vi "Empty_Complete.vi"(11 "input cluster":T1={"Pinch-valve"="Test Sample", "XLP 6000 Pump"="MRJ", "Camera1"="", "Camera2"="", "Img_Capt"=FALSE, "Actuator"=FALSE, "Pump"=FALSE, "Cam 1"=FALSE, "Cam 2"=FALSE, "Empty_Refill"=FALSE, "Crop"=FALSE, "Light intensity"=0, "Exposure Time"=0.0, "Sample Name"="", "Operator"="", "Calibration 1"=path "C:/Users/au540322/Desktop/IHS_Project/images/Debris/Debris_0/Debris_0_2019_06_01-23-32-49-686.PNG", "Calibration 2"=path "C:/Users/au540322/Desktop/IHS_Project/images/Debris/Debris_0/Debris_0_2019_06_01-23-32-49-686.PNG", "Framerate"=1, "Timeout Sample"=1, "Collection date"="", "Sample size threshold"=500, "Empty start"=500, "Command"="", "Station"="", "Species Name"="", "Other Notes"="", "Aperture"=enum."Item 3", "Image Process Queue Size"=100, "Image Save Queue Size"=0, "Overload threshold"=0, "Max Framerate"=0, "Rectangle 1"={"Left"=0, "Top"=0, "Right"=0, "Bottom"=0, "Rotation"=0.0}, "Rectangle 2"={"Left"=0, "Top"=100, "Right"=100, "Bottom"=0, "Rotation"=0.0}, "Detection Region %"=200.0, "Detect 1"=path "C:/Users/au540322/Desktop/IHS_Project/images/Debris/Debris_0/Debris_0_2019_06_01-23-32-49-686.PNG", "Detect 2"=path "C:/Users/au540322/Desktop/IHS_Project/images/Debris/Debris_0/Debris_0_2019_06_01-23-32-49-686.PNG", "Max large object threshold"=500, "Open(T)/Close(F)"=FALSE, "Img_Capt Begin"=FALSE, "Dispense Speed"=0, "Flush Size"=0, "Location"="", "Latitude"="", "Longitude"="", "Determiner"="", "Sex"="", "Camera1_Img"=refnum, "Camera2_Img"=refnum, "Img1_Orig_Disp"=refnum, "Img2_Orig_Disp"=refnum, "Img1_Orig_RGB"=refnum, "Img2_Orig_RGB"=refnum, "Blue_Plane_Extract"=refnum, "Subtracted_Plane"=refnum, "Img1_Binary"=refnum, "Img2_Binary"=refnum, "Crop_Mask"=refnum, "Img1_Save"=refnum, "Img2_Save"=refnum, "Img1_Cali_Full"=refnum, "Img2_Cali_Full"=refnum, "Img1_Cali_Detect"=refnum, "Img2_Cali_Detect"=refnum, "Cam 1 queue"=refnum, "Cam 2 queue"=refnum, "Cam 1 - save queue"=refnum, "Cam 2 - save queue"=refnum, "Overlay_Ring"=0, "SystemVersion"=0, "System Serial"="", "Legacy Cam Attributes"=FALSE, "Camera Orientation 1"="", "Camera Orientation 2"="", "Pixel to mm 1"=0.0, "Pixel to mm 2"=0.0, "CAM1 Model"=enum."a2A5328-15ucBAS", "CAM2 Model"=enum."a2A5328-15ucBAS", "Flush Insect"=FALSE, "Pump Size"=FALSE, "Barcode"="", "Phase3"=FALSE, "Mega F3"="", "Container nr."=0.0, "Flush Error"=TRUE, "Start System"=FALSE, "Size Interval"=0.0, "Mun. of containers"=0.0, "Sorting sys."=FALSE, "Initial size"=0.0} {"SystemVersion" items=["Standard", "XL"]; "Overlay_Ring" items=["Session Data", "Extended Setup", "Buffer", "Camera", "Dispenser", "Stats", "Connections"]; "Flush Size" min=1; "Dispense Speed" min=1; "Rectangle 2"."Rotation" format="%.2f"; "Rectangle 2"."Left" scale=0.0..1024.0; "Rectangle 2"."Right" scale=0.0..1024.0; "Rectangle 1"."Rotation" format="%.2f"; "Rectangle 1"."Left" scale=0.0..1024.0; "Rectangle 1"."Right" scale=0.0..1024.0; "Max Framerate" min=1; "Overload threshold" min=1; "Image Save Queue Size" min=1; "Image Process Queue Size" min=1; "Empty start" min=1; "Sample size threshold" min=1; "Framerate" min=1; "Light intensity" scale=0.0..100.0}) -> (0 "Next State":T5=enum."Pump Cycle", 3 "output cluster":T1={"Pinch-valve"="Test Sample", "XLP 6000 Pump"="MRJ", "Camera1"="", "Camera2"="", "Img_Capt"=FALSE, "Actuator"=FALSE, "Pump"=FALSE, "Cam 1"=FALSE, "Cam 2"=FALSE, "Empty_Refill"=FALSE, "Crop"=FALSE, "Light intensity"=0, "Exposure Time"=0.0, "Sample Name"="", "Operator"="", "Calibration 1"=path "C:/Users/au540322/Desktop/IHS_Project/images/Debris/Debris_0/Debris_0_2019_06_01-23-32-49-686.PNG", "Calibration 2"=path "C:/Users/au540322/Desktop/IHS_Project/images/Debris/Debris_0/Debris_0_2019_06_01-23-32-49-686.PNG", "Framerate"=100, "Timeout Sample"=500, "Collection date"="", "Sample size threshold"=500, "Empty start"=500, "Command"="", "Station"="", "Species Name"="", "Other Notes"="", "Aperture"=enum."Item 3", "Image Process Queue Size"=100, "Image Save Queue Size"=0, "Overload threshold"=0, "Max Framerate"=0, "Rectangle 1"={"Left"=0, "Top"=0, "Right"=0, "Bottom"=0, "Rotation"=0.0}, "Rectangle 2"={"Left"=0, "Top"=100, "Right"=100, "Bottom"=0, "Rotation"=0.0}, "Detection Region %"=200.0, "Detect 1"=path "C:/Users/au540322/Desktop/IHS_Project/images/Debris/Debris_0/Debris_0_2019_06_01-23-32-49-686.PNG", "Detect 2"=path "C:/Users/au540322/Desktop/IHS_Project/images/Debris/Debris_0/Debris_0_2019_06_01-23-32-49-686.PNG", "Max large object threshold"=500, "Open(T)/Close(F)"=FALSE, "Img_Capt Begin"=FALSE, "Dispense Speed"=0, "Flush Size"=0, "Location"="", "Latitude"="", "Longitude"="", "Determiner"="", "Sex"="", "Camera1_Img"=refnum, "Camera2_Img"=refnum, "Img1_Orig_Disp"=refnum, "Img2_Orig_Disp"=refnum, "Img1_Orig_RGB"=refnum, "Img2_Orig_RGB"=refnum, "Blue_Plane_Extract"=refnum, "Subtracted_Plane"=refnum, "Img1_Binary"=refnum, "Img2_Binary"=refnum, "Crop_Mask"=refnum, "Img1_Save"=refnum, "Img2_Save"=refnum, "Img1_Cali_Full"=refnum, "Img2_Cali_Full"=refnum, "Img1_Cali_Detect"=refnum, "Img2_Cali_Detect"=refnum, "Cam 1 queue"=refnum, "Cam 2 queue"=refnum, "Cam 1 - save queue"=refnum, "Cam 2 - save queue"=refnum, "Overlay_Ring"=0, "SystemVersion"=0, "System Serial"="", "Legacy Cam Attributes"=FALSE, "Camera Orientation 1"="", "Camera Orientation 2"="", "Pixel to mm 1"=0.0, "Pixel to mm 2"=0.0, "CAM1 Model"=enum."a2A5328-15ucBAS", "CAM2 Model"=enum."a2A5328-15ucBAS", "Flush Insect"=FALSE, "Pump Size"=FALSE, "Barcode"="", "Phase3"=FALSE, "Mega F3"="", "Container nr."=0.0, "Flush Error"=TRUE, "Start System"=FALSE, "Size Interval"=0.0, "Mun. of containers"=0.0, "Sorting sys."=FALSE, "Initial size"=0.0} {"SystemVersion" items=["Standard", "XL"]; "Overlay_Ring" items=["Session Data", "Extended Setup", "Buffer", "Camera", "Dispenser", "Stats", "Connections"]; "Flush Size" min=1; "Dispense Speed" min=1; "Rectangle 2"."Rotation" format="%.2f"; "Rectangle 2"."Left" scale=0.0..1024.0; "Rectangle 2"."Right" scale=0.0..1024.0; "Rectangle 1"."Rotation" format="%.2f"; "Rectangle 1"."Left" scale=0.0..1024.0; "Rectangle 1"."Right" scale=0.0..1024.0; "Max Framerate" min=1; "Overload threshold" min=1; "Image Save Queue Size" min=1; "Image Process Queue Size" min=1; "Empty start" min=1; "Sample size threshold" min=1; "Framerate" min=1; "Light intensity" scale=0.0..100.0})   [LabVIEW 2024]
uses:
  controls/Data.ctl
  <vilib>/userDefined/High Color/IMAQdx.ctl
  <vilib>/vision/Image Controls.llb/IMAQ Image.ctl
  controls/State.ctl
  50916f46-f414-496b-a007-128175b6596b.vi
  dc7e33f5-77bc-44ac-8d45-fe06c071e168.vi
  6ae0c342-c8b8-4515-b876-f0496a2b3108.vi
  52bd93dd-9142-4977-bffa-4dc7adc43fdc.vi
panel:
  out "VISA resource name out":refnum<visa-resource-name>
  out "error out":errorcluster
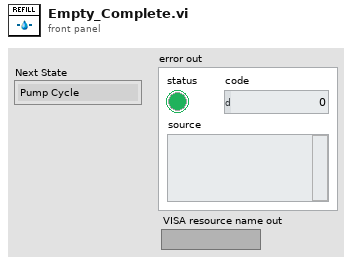
[diagram p1: front panel]
types:
  T1 = typedef "Data.ctl" = cluster{"Pinch-valve":refnum<visa-resource-name>, "XLP 6000 Pump":refnum<visa-resource-name>, "Camera1":T2, "Camera2":T2, "Img_Capt":bool, "Actuator":bool, "Pump":bool, "Cam 1":bool, "Cam 2":bool, "Empty_Refill":bool, "Crop":bool, "Light intensity":i32, "Exposure Time":dbl, "Sample Name":string, "Operator":string, "Calibration 1":path, "Calibration 2":path, "Framerate":i32, "Timeout Sample":i32, "Collection date":string, "Sample size threshold":i32, "Empty start":u32, "Command":string, "Station":string, "Species Name":string, "Other Notes":string, "Aperture":enum32{"Item 0", "Item 1", "Item 2", "Item 3"}, "Image Process Queue Size":i32, "Image Save Queue Size":i32, "Overload threshold":i32, "Max Framerate":i32, "Rectangle 1":T3, "Rectangle 2":T3, "Detection Region %":dbl, "Detect 1":path, "Detect 2":path, "Max large object threshold":i32, "Open(T)/Close(F)":bool, "Img_Capt Begin":bool, "Dispense Speed":i32, "Flush Size":i32, "Location":string, "Latitude":string, "Longitude":string, "Determiner":string, "Sex":string, "Camera1_Img":T4, "Camera2_Img":T4, "Img1_Orig_Disp":T4, "Img2_Orig_Disp":T4, "Img1_Orig_RGB":T4, "Img2_Orig_RGB":T4, "Blue_Plane_Extract":T4, "Subtracted_Plane":T4, "Img1_Binary":T4, "Img2_Binary":T4, "Crop_Mask":T4, "Img1_Save":T4, "Img2_Save":T4, "Img1_Cali_Full":T4, "Img2_Cali_Full":T4, "Img1_Cali_Detect":T4, "Img2_Cali_Detect":T4, "Cam 1 queue":refnum<queue>, "Cam 2 queue":refnum<queue>, "Cam 1 - save queue":refnum<queue>, "Cam 2 - save queue":refnum<queue>, "Overlay_Ring":u16, "SystemVersion":u16, "System Serial":string, "Legacy Cam Attributes":bool, "Camera Orientation 1":string, "Camera Orientation 2":string, "Pixel to mm 1":dbl, "Pixel to mm 2":dbl, "CAM1 Model":enum16{"a2A5328-15ucBAS", "acA1920-155uc"}, "CAM2 Model":enum16{"a2A5328-15ucBAS", "acA1920-155uc"}, "Flush Insect":bool, "Pump Size":bool, "Barcode":string, "Phase3":bool, "Mega F3":refnum<visa-resource-name>, "Container nr.":dbl, "Flush Error":bool, "Start System":bool, "Size Interval":dbl, "Mun. of containers":dbl, "Sorting sys.":bool, "Initial size":dbl}
  T2 = typedef "IMAQdx.ctl" = refnum<k21>
  T3 = typedef "IMAQ Rectangle" = cluster{"Left":i32, "Top":i32, "Right":i32, "Bottom":i32, "Rotation":dbl}
  T4 = typedef "IMAQ Image.ctl" = refnum<image>
  T5 = typedef "State.ctl" = enum16{"Initialize", "Wait for Event", "Position", "Valve Signal", "Extra Flush", "Valve Cycle", "Valve Open", "Valve Close", "Pump Command", "Pump Cycle", "Empty System", "Start System", "Connect Systems", "Start Image Capture", "Stop Image Capture", "Calibration Pictures", "StatusRequest", "RequestBarcodes", "SendBarcode", "ReturnHome", "ReInit. F3", "Clear F3 Error", "CursorIdle", "Exit"}
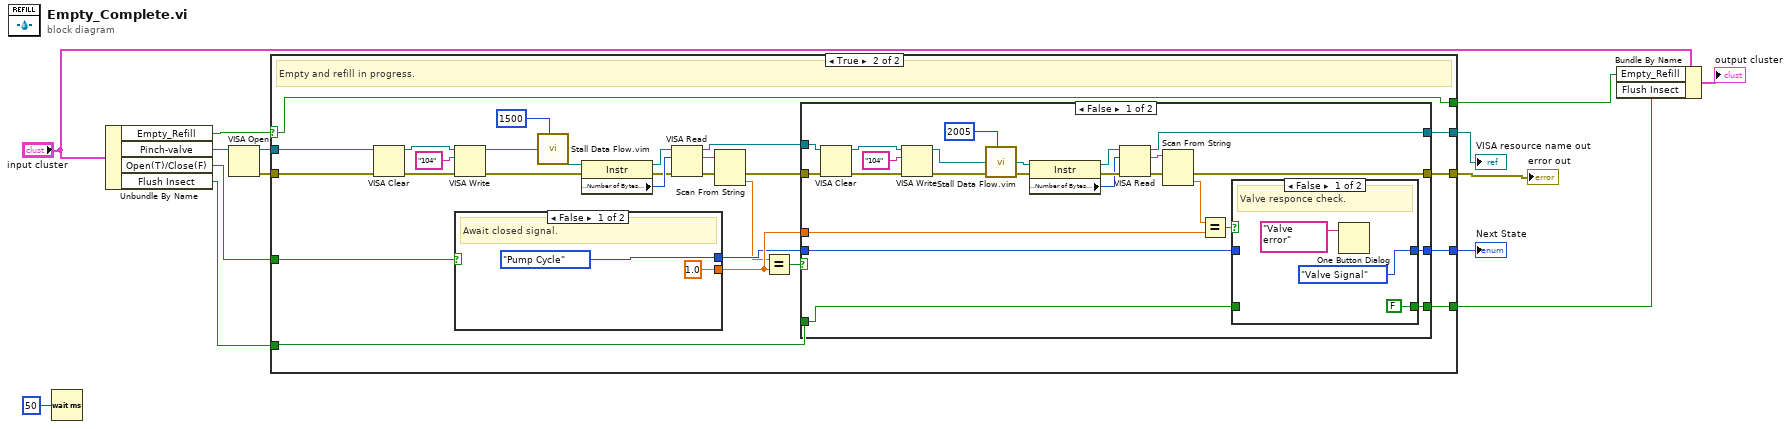
[diagram p0: block diagram]
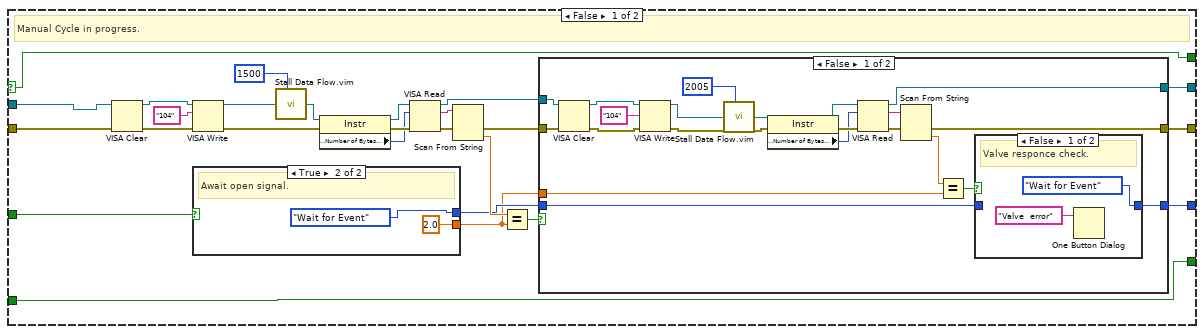
[diagram p2: hidden frame]
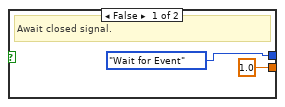
[diagram p5: hidden frame]
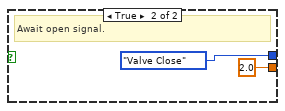
[diagram p8: hidden frame]
diagram:
  n1 = Wait (ms)(milliseconds to wait=u32 50) -> ()  [unwired: 1 out]
  n2 = Unbundle By Name("input cluster") -> ("Empty_Refill"=w14:bool, "Pinch-valve"=w13:refnum<visa-resource-name>, "Open(T)/Close(F)"=w7:bool, "Flush Insect"=w2:bool)
  n3 = VISA Open(VISA resource name=w13) -> (VISA resource name=w5:refnum<visa-resource-name>, error out=w6:errorcluster)  [unwired: 4 in]
  n4 = case shown="True" w14 {
    selector: w14 -> [w39 w83]
    tunnel: [w25 w80] -> w11
    tunnel: [w39 w83] -> w9
    tunnel: w7 -> [w40 w82]
    tunnel: [w19 w81] -> w4
    tunnel: w6 -> [w18 w75]
    tunnel: w5 -> [w16 w74]
    tunnel: [w17 w76] -> w3
    tunnel: w2 -> [w15 w72]
    tunnel: [w15 w73] -> w1
    frame False {
      # "Manual Cycle in progress."
      n5 = VISA Clear(VISA resource name=w16, error in (no error)=w18) -> (VISA resource name out=w38:refnum<visa-resource-name>, error out=w37:errorcluster)
      n6 = VISA Write(VISA resource name=w38, write buffer="104", error in (no error)=w37) -> (VISA resource name out=w31:refnum<visa-resource-name>, error out=w32:errorcluster)  [unwired: 1 out]
      n7 = case shown="True" w40 {
        tunnel: [State."Wait for Event" ("Next State") State."Wait for Event" ("Next State")] -> w26
        tunnel: [1.0 2.0] -> w23
        frame False {
          # "Await closed signal."
        }
        frame True {
          # "Await open signal."
        }
      }
      n8 = call "Stall Data Flow.vim"("value in"=w31, "milliseconds to wait"=u32 1500) -> ("value out"=w30:refnum<visa-resource-name>)  [unwired: 1 out]
      n9 = property class="Instr"(reference=w30, error in=w32) -> (reference out=w35:refnum<visa-resource-name>, error out=w34:errorcluster, "Serial Settings:Number of Bytes at Serial Port"=w33:u32)
      n10 = VISA Read(VISA resource name=w35, byte count=w33, error in (no error)=w34) -> (VISA resource name out=w24:refnum<visa-resource-name>, read buffer=w29:string, error out=w22:errorcluster)  [unwired: 1 out]
      n11 = Scan From String(input string=w29, error in=w22) -> (error out=w21:errorcluster, output 1=w28:dbl)  [unwired: 3 in, 2 out]
      n12 = Equal?(x=w28, y=w23) -> (x = y?=w27:bool)
      n13 = case shown="False" w27 {
        tunnel: w26 -> [w61 w67]
        tunnel: [w60 w67] -> w25
        tunnel: w24 -> [w44 w65]
        tunnel: w21 -> [w43 w66]
        tunnel: [w55 w65] -> w19
        tunnel: [w48 w66] -> w17
        tunnel: w23 -> [w50 _]
        frame False {
          n14 = VISA Clear(VISA resource name=w44, error in (no error)=w43) -> (VISA resource name out=w47:refnum<visa-resource-name>, error out=w46:errorcluster)
          n15 = VISA Write(VISA resource name=w47, write buffer="104", error in (no error)=w46) -> (VISA resource name out=w41:refnum<visa-resource-name>, error out=w42:errorcluster)  [unwired: 1 out]
          n16 = call "Stall Data Flow.vim"("value in"=w41, "milliseconds to wait"=u32 2005) -> ("value out"=w56:refnum<visa-resource-name>)  [unwired: 1 out]
          n17 = property class="Instr"(reference=w56, error in=w42) -> (reference out=w59:refnum<visa-resource-name>, error out=w58:errorcluster, "Serial Settings:Number of Bytes at Serial Port"=w57:u32)
          n18 = VISA Read(VISA resource name=w59, byte count=w57, error in (no error)=w58) -> (VISA resource name out=w55:refnum<visa-resource-name>, read buffer=w53:string, error out=w49:errorcluster)  [unwired: 1 out]
          n19 = Scan From String(input string=w53, error in=w49) -> (error out=w48:errorcluster, output 1=w51:dbl)  [unwired: 3 in, 2 out]
          n20 = Equal?(x=w51, y=w50) -> (x = y?=w52:bool)
          n21 = case shown="False" w52 {
            tunnel: [State."Wait for Event" ("Next State") w64] -> w60
            tunnel: w61 -> [_ w64]
            frame False {
              # "Valve responce check."
              n22 = One Button Dialog(message="Valve  error") -> ()  [unwired: 1 in, 1 out]
            }
            frame True {
              # "Valve responce check."
            }
          }
        }
        frame True {
        }
      }
    }
    frame True {
      # "Empty and refill in progress."
      n23 = VISA Clear(VISA resource name=w74, error in (no error)=w75) -> (VISA resource name out=w85:refnum<visa-resource-name>, error out=w86:errorcluster)
      n24 = VISA Write(VISA resource name=w85, write buffer="104", error in (no error)=w86) -> (VISA resource name out=w91:refnum<visa-resource-name>, error out=w90:errorcluster)  [unwired: 1 out]
      n25 = case shown="False" w82 {
        tunnel: [State."Pump Cycle" ("Next State") State."Valve Close" ("Next State")] -> w96
        tunnel: [1.0 2.0] -> w98
        frame False {
          # "Await closed signal."
        }
        frame True {
          # "Await open signal."
        }
      }
      n26 = call "Stall Data Flow.vim"("value in"=w91, "milliseconds to wait"=u32 1500) -> ("value out"=w92:refnum<visa-resource-name>)  [unwired: 1 out]
      n27 = property class="Instr"(reference=w92, error in=w90) -> (reference out=w87:refnum<visa-resource-name>, error out=w88:errorcluster, "Serial Settings:Number of Bytes at Serial Port"=w89:u32)
      n28 = VISA Read(VISA resource name=w87, byte count=w89, error in (no error)=w88) -> (VISA resource name out=w97:refnum<visa-resource-name>, read buffer=w93:string, error out=w79:errorcluster)  [unwired: 1 out]
      n29 = Scan From String(input string=w93, error in=w79) -> (error out=w78:errorcluster, output 1=w94:dbl)  [unwired: 3 in, 2 out]
      n30 = Equal?(x=w94, y=w98) -> (x = y?=w95:bool)
      n31 = case shown="False" w95 {
        tunnel: w96 -> [w121 w130]
        tunnel: [w120 w130] -> w80
        tunnel: w97 -> [w101 w128]
        tunnel: w78 -> [w104 w129]
        tunnel: [w115 w128] -> w81
        tunnel: [w108 w129] -> w76
        tunnel: w98 -> [w110 _]
        tunnel: w72 -> [w100 w127]
        tunnel: [w99 w127] -> w73
        frame False {
          n32 = VISA Clear(VISA resource name=w101, error in (no error)=w104) -> (VISA resource name out=w102:refnum<visa-resource-name>, error out=w103:errorcluster)
          n33 = VISA Write(VISA resource name=w102, write buffer="104", error in (no error)=w103) -> (VISA resource name out=w105:refnum<visa-resource-name>, error out=w106:errorcluster)  [unwired: 1 out]
          n34 = call "Stall Data Flow.vim"("value in"=w105, "milliseconds to wait"=u32 2005) -> ("value out"=w116:refnum<visa-resource-name>)  [unwired: 1 out]
          n35 = property class="Instr"(reference=w116, error in=w106) -> (reference out=w119:refnum<visa-resource-name>, error out=w118:errorcluster, "Serial Settings:Number of Bytes at Serial Port"=w117:u32)
          n36 = VISA Read(VISA resource name=w119, byte count=w117, error in (no error)=w118) -> (VISA resource name out=w115:refnum<visa-resource-name>, read buffer=w113:string, error out=w109:errorcluster)  [unwired: 1 out]
          n37 = Scan From String(input string=w113, error in=w109) -> (error out=w108:errorcluster, output 1=w111:dbl)  [unwired: 3 in, 2 out]
          n38 = Equal?(x=w111, y=w110) -> (x = y?=w112:bool)
          n39 = case shown="False" w112 {
            tunnel: [State."Valve Signal" ("Next State") w126] -> w120
            tunnel: w121 -> [_ w126]
            tunnel: w100 -> [_ w125]
            tunnel: [FALSE ("Flush Insect") w125] -> w99
            frame False {
              # "Valve responce check."
              n40 = One Button Dialog(message="Valve  error") -> ()  [unwired: 1 in, 1 out]
            }
            frame True {
              # "Valve responce check."
            }
          }
        }
        frame True {
        }
      }
    }
  }
  "Next State" <- w11
  "error out" <- w3
  "VISA resource name out" <- w4
  n41 = Bundle By Name(cluster="input cluster", "Empty_Refill"=w9, "Flush Insect"=w1) -> (→"output cluster":T1)
